vi "S4GUI.vi"() -> ()   [LabVIEW 2018] (continued)
  T9 = cluster{"Trigger Mode Status":string, "String output":string, "Instrument Status":cluster{"WPROT pos":dbl, "WPSEL pos":dbl, "GMIR pos":dbl, "GFOC pos":dbl, "CALW pos":dbl, "ASEL pos":dbl, "connection":bool, "mode":bool, "String Status":string}, "Sync Box State":i32, "Trigger General Status":string, "Instrument States":cluster{"WPSEL State":i32, "WPROT State":i32, "CALW State":i32, "ASEL State":i32, "GMIR State":i32, "GFOC State":i32}, "Instrument Pos Names":cluster{"WPROT posname":string, "WPSEL posname":string, "CALW posname":string, "ASEL posname":string}, "ChannelA_Status":cluster{"Current exp":dbl, "Frames done":u32, "LastFileImage":string, "CamStatus":string, "Run state":u32, "connection":bool, "Cooler ON/OFF":i16, "Currently temperature":i16, "Temperature Status":string, "target  temp":i16, "conf runing":bool}, "WPROT seq":u16, "ChannelB_Status":cluster{"Current exp":dbl, "Frames done":u32, "LastFileImage":string, "CamStatus":string, "Run state":u32, "connection":bool, "Cooler ON/OFF":i16, "Currently temperature":i16, "Temperature Status":string, "target  temp":i16, "conf runing":bool}, "ChannelC_Status":cluster{"Current exp":dbl, "Frames done":u32, "LastFileImage":string, "CamStatus":string, "Run state":u32, "connection":bool, "Cooler ON/OFF":i16, "Currently temperature":i16, "Temperature Status":string, "target  temp":i16, "conf runing":bool}, "ChannelD_Status":cluster{"Current exp":dbl, "Frames done":u32, "LastFileImage":string, "CamStatus":string, "Run state":u32, "connection":bool, "Cooler ON/OFF":i16, "Currently temperature":i16, "Temperature Status":string, "target  temp":i16, "conf runing":bool}, "ChannelA_CCD":cluster{"ACQUISITION_MODE":u8, "TRIGGER_MODE":u8, "READ_MODE":u8, "PREAMP":u8, "READOUT_RATE":u8, "VERTICAL_SHIFT_SPEED":u8, "EM_MODE":u8, "EM_GAIN":u16, "SHUTTER_MODE":u8, "SHUTTER_TTL":u8, "SHUTTER_OPENNING_TIME":u16, "SHUTTER_CLOSING_TIME":u16, "VBIN":u16, "HBIN":u16, "INITIAL_LINE":u16, "INITIAL_COLUMN":u16, "FINAL_LINE":u16, "FINAL_COLUMN":u16, "FRAME_TRANSFER":bool, "VERTICAL_CLOCK_VOLTAGE":u8, "AD_CHANNEL":u32}, "ChannelB_CCD ":cluster{"ACQUISITION_MODE":u8, "TRIGGER_MODE":u8, "READ_MODE":u8, "PREAMP":u8, "READOUT_RATE":u8, "VERTICAL_SHIFT_SPEED":u8, "EM_MODE":u8, "EM_GAIN":u16, "SHUTTER_MODE":u8, "SHUTTER_TTL":u8, "SHUTTER_OPENNING_TIME":u16, "SHUTTER_CLOSING_TIME":u16, "VBIN":u16, "HBIN":u16, "INITIAL_LINE":u16, "INITIAL_COLUMN":u16, "FINAL_LINE":u16, "FINAL_COLUMN":u16, "FRAME_TRANSFER":bool, "VERTICAL_CLOCK_VOLTAGE":u8, "AD_CHANNEL":u32}, "ChannelC_CCD":cluster{"ACQUISITION_MODE":u8, "TRIGGER_MODE":u8, "READ_MODE":u8, "PREAMP":u8, "READOUT_RATE":u8, "VERTICAL_SHIFT_SPEED":u8, "EM_MODE":u8, "EM_GAIN":u16, "SHUTTER_MODE":u8, "SHUTTER_TTL":u8, "SHUTTER_OPENNING_TIME":u16, "SHUTTER_CLOSING_TIME":u16, "VBIN":u16, "HBIN":u16, "INITIAL_LINE":u16, "INITIAL_COLUMN":u16, "FINAL_LINE":u16, "FINAL_COLUMN":u16, "FRAME_TRANSFER":bool, "VERTICAL_CLOCK_VOLTAGE":u8, "AD_CHANNEL":u32}, "ChannelD_CCD":cluster{"ACQUISITION_MODE":u8, "TRIGGER_MODE":u8, "READ_MODE":u8, "PREAMP":u8, "READOUT_RATE":u8, "VERTICAL_SHIFT_SPEED":u8, "EM_MODE":u8, "EM_GAIN":u16, "SHUTTER_MODE":u8, "SHUTTER_TTL":u8, "SHUTTER_OPENNING_TIME":u16, "SHUTTER_CLOSING_TIME":u16, "VBIN":u16, "HBIN":u16, "INITIAL_LINE":u16, "INITIAL_COLUMN":u16, "FINAL_LINE":u16, "FINAL_COLUMN":u16, "FRAME_TRANSFER":bool, "VERTICAL_CLOCK_VOLTAGE":u8, "AD_CHANNEL":u32}, "CHA_Checked Params":cluster{"ACQUISITION_MODE":bool, "TRIGGER_MODE":bool, "READ_MODE":bool, "PREAMP":bool, "READOUT_RATE":bool, "VERTICAL_SHIFT_SPEED":bool, "EM_MODE":bool, "EM_GAIN":bool, "SHUTTER_MODE":bool, "SHUTTER_TTL":bool, "SHUTTER_OPENING_TIME":bool, "SHUTTER_CLOSING_TIME":bool, "VBIN":bool, "HBIN":bool, "INITIAL_LINE":bool, "INITIAL_COLUMN":bool, "FINAL_LINE":bool, "FINAL_COLUMN":bool, "FRAME_TRANSFER":bool, "VERTICAL_CLOCK_VOLTAGE":bool, "AD_CHANNEL":bool}, "CHB_Checked Params":cluster{"ACQUISITION_MODE":bool, "TRIGGER_MODE":bool, "READ_MODE":bool, "PREAMP":bool, "READOUT_RATE":bool, "VERTICAL_SHIFT_SPEED":bool, "EM_MODE":bool, "EM_GAIN":bool, "SHUTTER_MODE":bool, "SHUTTER_TTL":bool, "SHUTTER_OPENING_TIME":bool, "SHUTTER_CLOSING_TIME":bool, "VBIN":bool, "HBIN":bool, "INITIAL_LINE":bool, "INITIAL_COLUMN":bool, "FINAL_LINE":bool, "FINAL_COLUMN":bool, "FRAME_TRANSFER":bool, "VERTICAL_CLOCK_VOLTAGE":bool, "AD_CHANNEL":bool}, "CHC_Checked Params":cluster{"ACQUISITION_MODE":bool, "TRIGGER_MODE":bool, "READ_MODE":bool, "PREAMP":bool, "READOUT_RATE":bool, "VERTICAL_SHIFT_SPEED":bool, "EM_MODE":bool, "EM_GAIN":bool, "SHUTTER_MODE":bool, "SHUTTER_TTL":bool, "SHUTTER_OPENING_TIME":bool, "SHUTTER_CLOSING_TIME":bool, "VBIN":bool, "HBIN":bool, "INITIAL_LINE":bool, "INITIAL_COLUMN":bool, "FINAL_LINE":bool, "FINAL_COLUMN":bool, "FRAME_TRANSFER":bool, "VERTICAL_CLOCK_VOLTAGE":bool, "AD_CHANNEL":bool}, "CHD_Checked Params":cluster{"ACQUISITION_MODE":bool, "TRIGGER_MODE":bool, "READ_MODE":bool, "PREAMP":bool, "READOUT_RATE":bool, "VERTICAL_SHIFT_SPEED":bool, "EM_MODE":bool, "EM_GAIN":bool, "SHUTTER_MODE":bool, "SHUTTER_TTL":bool, "SHUTTER_OPENING_TIME":bool, "SHUTTER_CLOSING_TIME":bool, "VBIN":bool, "HBIN":bool, "INITIAL_LINE":bool, "INITIAL_COLUMN":bool, "FINAL_LINE":bool, "FINAL_COLUMN":bool, "FRAME_TRANSFER":bool, "VERTICAL_CLOCK_VOLTAGE":bool, "AD_CHANNEL":bool}, "Trigger_connection":bool, "TCSPD_connection":bool, "TCS extended":string}
  T10 = cluster{"Cluster Mode Sync":cluster{"#Index Cycles":enum8{"Enabled", "Disabled", "Disabled and Grayed Out"}, "#Cycles":enum8{"Enabled", "Disabled", "Disabled and Grayed Out"}, "SSM":enum8{"Enabled", "Disabled", "Disabled and Grayed Out"}, "Set SM":enum8{"Enabled", "Disabled", "Disabled and Grayed Out"}, "Star SM":enum8{"Enabled", "Disabled", "Disabled and Grayed Out"}, "Pause SM":enum8{"Enabled", "Disabled", "Disabled and Grayed Out"}, "Stop SM":enum8{"Enabled", "Disabled", "Disabled and Grayed Out"}, "Abort SM":enum8{"Enabled", "Disabled", "Disabled and Grayed Out"}, "Start SM Text":string}, "Cluster Polarimetry":cluster{"Lambda Selector":enum8{"Enabled", "Disabled", "Disabled and Grayed Out"}, "Calibrator Selector":enum8{"Enabled", "Disabled", "Disabled and Grayed Out"}, "Set Waveplate":enum8{"Enabled", "Disabled", "Disabled and Grayed Out"}, "Select Positions":enum8{"Enabled", "Disabled", "Disabled and Grayed Out"}, "P0":enum8{"Enabled", "Disabled", "Disabled and Grayed Out"}, "P1":enum8{"Enabled", "Disabled", "Disabled and Grayed Out"}, "P2":enum8{"Enabled", "Disabled", "Disabled and Grayed Out"}, "P3":enum8{"Enabled", "Disabled", "Disabled and Grayed Out"}, "P4":enum8{"Enabled", "Disabled", "Disabled and Grayed Out"}, "P5":enum8{"Enabled", "Disabled", "Disabled and Grayed Out"}, "P6":enum8{"Enabled", "Disabled", "Disabled and Grayed Out"}, "P7":enum8{"Enabled", "Disabled", "Disabled and Grayed Out"}, "P8":enum8{"Enabled", "Disabled", "Disabled and Grayed Out"}, "P9":enum8{"Enabled", "Disabled", "Disabled and Grayed Out"}, "P10":enum8{"Enabled", "Disabled", "Disabled and Grayed Out"}, "P11":enum8{"Enabled", "Disabled", "Disabled and Grayed Out"}, "P12":enum8{"Enabled", "Disabled", "Disabled and Grayed Out"}, "P13":enum8{"Enabled", "Disabled", "Disabled and Grayed Out"}, "P14":enum8{"Enabled", "Disabled", "Disabled and Grayed Out"}, "P15":enum8{"Enabled", "Disabled", "Disabled and Grayed Out"}}, "Cluster Mode CH1":cluster{"#cycles ch1":enum8{"Enabled", "Disabled", "Disabled and Grayed Out"}, "Start ch1":enum8{"Enabled", "Disabled", "Disabled and Grayed Out"}, "Pause ch1":enum8{"Enabled", "Disabled", "Disabled and Grayed Out"}, "Stop ch1":enum8{"Enabled", "Disabled", "Disabled and Grayed Out"}, "Abort ch1":enum8{"Enabled", "Disabled", "Disabled and Grayed Out"}, "Exptime ch1":enum8{"Enabled", "Disabled", "Disabled and Grayed Out"}, "Exp ch1":enum8{"Enabled", "Disabled", "Disabled and Grayed Out"}, "Start ch1 Text":string, "Set Cooler":enum8{"Enabled", "Disabled", "Disabled and Grayed Out"}, "Set Temp":enum8{"Enabled", "Disabled", "Disabled and Grayed Out"}}, "Cluster Mode CH2":cluster{"#cycles ch2":enum8{"Enabled", "Disabled", "Disabled and Grayed Out"}, "Start ch2":enum8{"Enabled", "Disabled", "Disabled and Grayed Out"}, "Pause ch2":enum8{"Enabled", "Disabled", "Disabled and Grayed Out"}, "Stop ch2":enum8{"Enabled", "Disabled", "Disabled and Grayed Out"}, "Abort ch2":enum8{"Enabled", "Disabled", "Disabled and Grayed Out"}, "Exptime ch2":enum8{"Enabled", "Disabled", "Disabled and Grayed Out"}, "Exp ch2":enum8{"Enabled", "Disabled", "Disabled and Grayed Out"}, "Start ch2 Text":string, "Set Cooler":enum8{"Enabled", "Disabled", "Disabled and Grayed Out"}, "Set Temp":enum8{"Enabled", "Disabled", "Disabled and Grayed Out"}}, "Cluster Mode CH3":cluster{"#cycles ch3":enum8{"Enabled", "Disabled", "Disabled and Grayed Out"}, "Start ch3":enum8{"Enabled", "Disabled", "Disabled and Grayed Out"}, "Pause ch3":enum8{"Enabled", "Disabled", "Disabled and Grayed Out"}, "Stop ch3":enum8{"Enabled", "Disabled", "Disabled and Grayed Out"}, "Abort ch3":enum8{"Enabled", "Disabled", "Disabled and Grayed Out"}, "Exptime ch3":enum8{"Enabled", "Disabled", "Disabled and Grayed Out"}, "Exp ch3":enum8{"Enabled", "Disabled", "Disabled and Grayed Out"}, "Start ch3 Text":string, "Set Cooler":enum8{"Enabled", "Disabled", "Disabled and Grayed Out"}, "Set Temp":enum8{"Enabled", "Disabled", "Disabled and Grayed Out"}}, "Cluster Mode CH4":cluster{"#cycles ch4":enum8{"Enabled", "Disabled", "Disabled and Grayed Out"}, "Start ch4":enum8{"Enabled", "Disabled", "Disabled and Grayed Out"}, "Pause ch4":enum8{"Enabled", "Disabled", "Disabled and Grayed Out"}, "Stop ch4":enum8{"Enabled", "Disabled", "Disabled and Grayed Out"}, "Abort ch4":enum8{"Enabled", "Disabled", "Disabled and Grayed Out"}, "Exptime ch4":enum8{"Enabled", "Disabled", "Disabled and Grayed Out"}, "Exp ch4":enum8{"Enabled", "Disabled", "Disabled and Grayed Out"}, "Start ch4 Text":string, "Set Cooler":enum8{"Enabled", "Disabled", "Disabled and Grayed Out"}, "Set Temp":enum8{"Enabled", "Disabled", "Disabled and Grayed Out"}}, "Cluster ExpMode":cluster{"tab4":enum8{"Enabled", "Disabled", "Disabled and Grayed Out"}}}
  T11 = cluster{"WPROT pos":dbl, "WPSEL pos":dbl, "GMIR pos":dbl, "GFOC pos":dbl, "CALW pos":dbl, "ASEL pos":dbl, "connection":bool, "mode":bool, "String Status":string}
  T12 = cluster{"WPSEL State":i32, "WPROT State":i32, "CALW State":i32, "ASEL State":i32, "GMIR State":i32, "GFOC State":i32}
  T13 = cluster{"WPROT posname":string, "WPSEL posname":string, "CALW posname":string, "ASEL posname":string}
  T14 = cluster{"Current exp":dbl, "Frames done":u32, "LastFileImage":string, "CamStatus":string, "Run state":u32, "connection":bool, "Cooler ON/OFF":i16, "Currently temperature":i16, "Temperature Status":string, "target  temp":i16, "conf runing":bool}
  T15 = cluster{"Lambda Selector":enum8{"Enabled", "Disabled", "Disabled and Grayed Out"}, "Calibrator Selector":enum8{"Enabled", "Disabled", "Disabled and Grayed Out"}, "Set Waveplate":enum8{"Enabled", "Disabled", "Disabled and Grayed Out"}, "Select Positions":enum8{"Enabled", "Disabled", "Disabled and Grayed Out"}, "P0":enum8{"Enabled", "Disabled", "Disabled and Grayed Out"}, "P1":enum8{"Enabled", "Disabled", "Disabled and Grayed Out"}, "P2":enum8{"Enabled", "Disabled", "Disabled and Grayed Out"}, "P3":enum8{"Enabled", "Disabled", "Disabled and Grayed Out"}, "P4":enum8{"Enabled", "Disabled", "Disabled and Grayed Out"}, "P5":enum8{"Enabled", "Disabled", "Disabled and Grayed Out"}, "P6":enum8{"Enabled", "Disabled", "Disabled and Grayed Out"}, "P7":enum8{"Enabled", "Disabled", "Disabled and Grayed Out"}, "P8":enum8{"Enabled", "Disabled", "Disabled and Grayed Out"}, "P9":enum8{"Enabled", "Disabled", "Disabled and Grayed Out"}, "P10":enum8{"Enabled", "Disabled", "Disabled and Grayed Out"}, "P11":enum8{"Enabled", "Disabled", "Disabled and Grayed Out"}, "P12":enum8{"Enabled", "Disabled", "Disabled and Grayed Out"}, "P13":enum8{"Enabled", "Disabled", "Disabled and Grayed Out"}, "P14":enum8{"Enabled", "Disabled", "Disabled and Grayed Out"}, "P15":enum8{"Enabled", "Disabled", "Disabled and Grayed Out"}}
  T16 = cluster{"#Index Cycles":enum8{"Enabled", "Disabled", "Disabled and Grayed Out"}, "#Cycles":enum8{"Enabled", "Disabled", "Disabled and Grayed Out"}, "SSM":enum8{"Enabled", "Disabled", "Disabled and Grayed Out"}, "Set SM":enum8{"Enabled", "Disabled", "Disabled and Grayed Out"}, "Star SM":enum8{"Enabled", "Disabled", "Disabled and Grayed Out"}, "Pause SM":enum8{"Enabled", "Disabled", "Disabled and Grayed Out"}, "Stop SM":enum8{"Enabled", "Disabled", "Disabled and Grayed Out"}, "Abort SM":enum8{"Enabled", "Disabled", "Disabled and Grayed Out"}, "Start SM Text":string}
  T17 = cluster{"#cycles ch1":enum8{"Enabled", "Disabled", "Disabled and Grayed Out"}, "Start ch1":enum8{"Enabled", "Disabled", "Disabled and Grayed Out"}, "Pause ch1":enum8{"Enabled", "Disabled", "Disabled and Grayed Out"}, "Stop ch1":enum8{"Enabled", "Disabled", "Disabled and Grayed Out"}, "Abort ch1":enum8{"Enabled", "Disabled", "Disabled and Grayed Out"}, "Exptime ch1":enum8{"Enabled", "Disabled", "Disabled and Grayed Out"}, "Exp ch1":enum8{"Enabled", "Disabled", "Disabled and Grayed Out"}, "Start ch1 Text":string, "Set Cooler":enum8{"Enabled", "Disabled", "Disabled and Grayed Out"}, "Set Temp":enum8{"Enabled", "Disabled", "Disabled and Grayed Out"}}
  T18 = cluster{"#cycles ch2":enum8{"Enabled", "Disabled", "Disabled and Grayed Out"}, "Start ch2":enum8{"Enabled", "Disabled", "Disabled and Grayed Out"}, "Pause ch2":enum8{"Enabled", "Disabled", "Disabled and Grayed Out"}, "Stop ch2":enum8{"Enabled", "Disabled", "Disabled and Grayed Out"}, "Abort ch2":enum8{"Enabled", "Disabled", "Disabled and Grayed Out"}, "Exptime ch2":enum8{"Enabled", "Disabled", "Disabled and Grayed Out"}, "Exp ch2":enum8{"Enabled", "Disabled", "Disabled and Grayed Out"}, "Start ch2 Text":string, "Set Cooler":enum8{"Enabled", "Disabled", "Disabled and Grayed Out"}, "Set Temp":enum8{"Enabled", "Disabled", "Disabled and Grayed Out"}}
  T19 = cluster{"#cycles ch3":enum8{"Enabled", "Disabled", "Disabled and Grayed Out"}, "Start ch3":enum8{"Enabled", "Disabled", "Disabled and Grayed Out"}, "Pause ch3":enum8{"Enabled", "Disabled", "Disabled and Grayed Out"}, "Stop ch3":enum8{"Enabled", "Disabled", "Disabled and Grayed Out"}, "Abort ch3":enum8{"Enabled", "Disabled", "Disabled and Grayed Out"}, "Exptime ch3":enum8{"Enabled", "Disabled", "Disabled and Grayed Out"}, "Exp ch3":enum8{"Enabled", "Disabled", "Disabled and Grayed Out"}, "Start ch3 Text":string, "Set Cooler":enum8{"Enabled", "Disabled", "Disabled and Grayed Out"}, "Set Temp":enum8{"Enabled", "Disabled", "Disabled and Grayed Out"}}
  T20 = cluster{"#cycles ch4":enum8{"Enabled", "Disabled", "Disabled and Grayed Out"}, "Start ch4":enum8{"Enabled", "Disabled", "Disabled and Grayed Out"}, "Pause ch4":enum8{"Enabled", "Disabled", "Disabled and Grayed Out"}, "Stop ch4":enum8{"Enabled", "Disabled", "Disabled and Grayed Out"}, "Abort ch4":enum8{"Enabled", "Disabled", "Disabled and Grayed Out"}, "Exptime ch4":enum8{"Enabled", "Disabled", "Disabled and Grayed Out"}, "Exp ch4":enum8{"Enabled", "Disabled", "Disabled and Grayed Out"}, "Start ch4 Text":string, "Set Cooler":enum8{"Enabled", "Disabled", "Disabled and Grayed Out"}, "Set Temp":enum8{"Enabled", "Disabled", "Disabled and Grayed Out"}}
  T21 = cluster{"ACQUISITION_MODE":u8, "TRIGGER_MODE":u8, "READ_MODE":u8, "PREAMP":u8, "READOUT_RATE":u8, "VERTICAL_SHIFT_SPEED":u8, "EM_MODE":u8, "EM_GAIN":u16, "SHUTTER_MODE":u8, "SHUTTER_TTL":u8, "SHUTTER_OPENNING_TIME":u16, "SHUTTER_CLOSING_TIME":u16, "VBIN":u16, "HBIN":u16, "INITIAL_LINE":u16, "INITIAL_COLUMN":u16, "FINAL_LINE":u16, "FINAL_COLUMN":u16, "FRAME_TRANSFER":bool, "VERTICAL_CLOCK_VOLTAGE":u8, "AD_CHANNEL":u32}
  T22 = cluster{"ACQUISITION_MODE":bool, "TRIGGER_MODE":bool, "READ_MODE":bool, "PREAMP":bool, "READOUT_RATE":bool, "VERTICAL_SHIFT_SPEED":bool, "EM_MODE":bool, "EM_GAIN":bool, "SHUTTER_MODE":bool, "SHUTTER_TTL":bool, "SHUTTER_OPENING_TIME":bool, "SHUTTER_CLOSING_TIME":bool, "VBIN":bool, "HBIN":bool, "INITIAL_LINE":bool, "INITIAL_COLUMN":bool, "FINAL_LINE":bool, "FINAL_COLUMN":bool, "FRAME_TRANSFER":bool, "VERTICAL_CLOCK_VOLTAGE":bool, "AD_CHANNEL":bool}
  T23 = cluster{"Image \nInitial Line":u16, "Image\nInitial Column":u16, "Image\nFinal Line":u16, "Image\nFInal Column":u16, "Vertical\nBinning":u16, "Horizontal\nBinning":u16, "Pre-amplification\nGain":u8, "CCD\nEM Gain":u16, "Readout\nRate":u8, "Shutter\nOpenning Time":i32, "Shutter\nClosing Time":i32, "Vertical\nShift Speed":u8, "Read\nMode":u8, "Vertical\nClock Voltage":u8, "A/D \nChannel":u32, "Shutter\nMode":u16, "Shutter\nTTL":u16, "Trigger\nMode":u16, "Frame\nTransfer":bool, "Acquisition\nMode":u8, "CCD \nEM Mode":u8}
  T24 = cluster{"ACQUISITION_MODE":u8, "TRIGGER_MODE":u8, "READ_MODE":u8, "PREAMP":u8, "READOUT_RATE":u8, "VERTICAL_SHIFT_SPEED":u8, "EM_MODE":u8, "EM_GAIN":u16, "SHUTTER_MODE":u8, "SHUTTER_TTL":u8, "SHUTTER_OPENING_TIME":u16, "SHUTTER_CLOSING_TIME":u16, "VBIN":u16, "HBIN":u16, "INITIAL_LINE":u16, "INITIAL_COLUMN":u16, "FINAL_LINE":u16, "FINAL_COLUMN":u16, "FRAME_TRANSFER":bool, "VERTICAL_CLOCK_VOLTAGE":u8, "AD_CHANNEL":u32}
  T25 = cluster{"Image Initial Line":dbl, "Image Initial Column":dbl, "Image Final Line":dbl, "Image FInal Column":dbl, "Vertical Binning":dbl, "Horizontal Binning":dbl, "Pre-amplification Gain":u8, "CCD EM Gain":u8, "Readout Rate":u8, "Shutter Openning Time":i32, "Shutter Closing Time":i32, "Vertical Shift Speed":u8, "Read Mode":u8, "Vertical Clock Voltage":u8, "A/D  Channel":u32, "Image Initial Line 2":dbl, "Image Initial Column 2":dbl, "Image Final Line 2":dbl, "Image FInal Column 2":dbl, "Vertical Binning 2":dbl, "Horizontal Binning 2":dbl, "Pre-amplification Gain 2":u8, "CCD EM Gain 2":u16, "Readout Rate 2":u8, "Shutter Openning Time 2":i32, "Shutter Closing Time 2":i32, "Vertical Shift Speed 2":u8, "Read Mode 2":u8, "Vertical Clock Voltage 2":u8, "A/D Channel 2":u32, "Image Initial Line 3":dbl, "Image Initial Column 3":dbl, "Image Final Line 3":dbl, "Image FInal Column 3":dbl, "Vertical Binning 3":dbl, "Horizontal Binning 3":dbl, "Pre-amplification Gain 3":u8, "CCD EM Gain 3":u16, "Readout Rate 3":u8, "Shutter Openning Time 3":i32, "Shutter Closing Time 3":i32, "Vertical Shift Speed 3":u8, "Read Mode 3":u8, "Vertical Clock Voltage 3":u8, "A/D Channel 3":u32, "Image Initial Line 4":dbl, "Image Initial Column 4":dbl, "Image Final Line 4":dbl, "Image FInal Column 4":dbl, "Vertical Binning 4":dbl, "Horizontal Binning 4":dbl, "Pre-amplification Gain 4":u8, "CCD EM Gain 4":u16, "Readout Rate 4":u8, "Shutter Openning Time 4":i32, "Shutter Closing Time 4":i32, "Vertical Shift Speed 4":u8, "Read Mode 4":u8, "Vertical Clock Voltage 4":u8, "A/D Channel 4":u32, "CCD EM Mode 2":u8, "CCD EM Mode 3":u8, "CCD EM Mode 4":u8, "CCD EM Mode":u16, "Shutter Mode":u16, "Shutter Mode 2":u16, "Shutter Mode 4":u16, "Shutter Mode 3":u16, "Shutter TTL":u16, "Shutter TTL 2":u16, "Shutter TTL 3":u16, "Shutter TTL 4":u16, "Frame Transfer":bool, "Frame Transfer 2":bool, "Frame Transfer 3":bool, "Frame Transfer 4":bool, "Trigger Mode":u16, "Trigger Mode 2":u16, "Trigger Mode 3":u16, "Trigger Mode 4":u16, "Acquisition Mode":u8, "Acquisition Mode 2":u8, "Acquisition Mode 3":u8, "Acquisition Mode 4":u8}
diagram:
  w5 = T7."Disabled" ("Disabled")
  (unwired) -400 ("Position:Top")
  w10 = "" ("Temp Status 1")
  w11 = i16 0 ("Curr Temp 1")
  w12 = FALSE ("Cooler status 1")
  w13 = u16 1 items=["Asynchronous", "Synchronous by Cycle"] ("SSM")
  (unwired) -400 ("Position:Top")
  w25 = u16 4 items=["All 16 positions", "First 8 positions", "First 4 positions", "1-4 & 9-12", "Clear", "Customized"] ("Select Positions")
  w4 = FALSE
  n1 = local write "Select Positions"(w25) -> ()
  n2 = property on="Tab Acq Type" class="TabCtl (strict)"("DisabledEnum"=T7."Disabled and Grayed Out" ("Disabled")) -> ()  [unwired: 2 in, 2 out]
  n3 = property on="Tab ObsEng" class="TabCtl (strict)"("Visible"=TRUE) -> ()  [unwired: 2 in, 2 out]
  n4 = flat-sequence {
    tunnel: errorcluster {"status"=FALSE, "code"=0, "source"=""} ("error in (no error)") -> [w30]
    tunnel: [w30] -> w7
    frame #0 {
      w31 = u32 240 ("Tab Control Pane Dimension:Width")
      w32 = u32 300 ("Tab Control Pane Dimension:Height")
      n5 = property on="Tab CH2" class="TabCtl (strict)"("PaneHeight"=w32, "PaneWidth"=w31) -> ()  [unwired: 2 in, 2 out]
      n6 = property on="Tab CH1" class="TabCtl (strict)"("PaneHeight"=w32, "PaneWidth"=w31) -> ()  [unwired: 2 in, 2 out]
      n7 = property on="Tab CH3" class="TabCtl (strict)"("PaneHeight"=w32, "PaneWidth"=w31) -> ()  [unwired: 2 in, 2 out]
      n8 = property on="Tab CH4" class="TabCtl (strict)"("PaneHeight"=w32, "PaneWidth"=w31) -> ()  [unwired: 2 in, 2 out]
      n9 = local write "loop max(ms)"(u32 0 ("loop max(ms)")) -> ()
    }
  }
  n10 = property on="SSM" class="Ring (strict)"("Value"=w13) -> ()  [unwired: 2 in, 2 out]
  n11 = disable-structure shown="Enabled" {
    disable-tunnel: "S4ACS_GUI.lvclass" -> [w41 w42]
    disable-tunnel: [w38 w42] -> w16
    disable-tunnel: w7 -> [w40 w43]
    disable-tunnel: [w39 w43] -> w15
    frame Enabled {
      # "Carrega o ultimo filtro escolhido para os 4 canais."
      n12 = local read "Filter1"() -> (w37:u8)
      n13 = local read "Filter2"() -> (w36:u8)
      n14 = local read "Filter3"() -> (w35:u8)
      n15 = local read "Filter4"() -> (w34:u8)
      n16 = call-dynamic "LoadFilters.vi"("Filter 4"=w34, "Filter 3"=w35, "error in (no error)"=w40, "Filter 2"=w36, "Filter 1"=w37, "S4GUI in"=w41) -> ("error out"=w39:errorcluster, "S4GUI out"=w38:refnum<class "S4GUI.lvclass">)  [unwired: 4 in]
    }
    frame Disabled {
    }
  }
  n17 = flat-sequence "Indicadores dos canais da parte inferior da tela principal" {
    frame #0 {
      w44 = ""
      "B1" <- w44
      "PA1" <- w44
      "RO1" <- w44
      "G1" <- w44
      "SI2" <- w44
      "PA2" <- w44
      "G2" <- w44
      "B2" <- w44
      "RO2" <- w44
      "EA2" <- w44
      "SI3" <- w44
      "EA3" <- w44
      "PA3" <- w44
      "B3" <- w44
      "G3" <- w44
      "RO3" <- w44
      "SI4" <- w44
      "EA4" <- w44
      "PA4" <- w44
      "B4" <- w44
      "G4" <- w44
      "RO4" <- w44
      "SI1" <- w44
      "EA1" <- w44
    }
  }
  n18 = local write "Cooler status 4"(w12) -> ()
  n19 = local write "Curr Temp 4"(w11) -> ()
  n20 = local write "Panel Temp 4"(w11) -> ()
  n21 = local write "Temp Status 4"(w10) -> ()
  n22 = local write "Panel cooler 4"(w12) -> ()
  n23 = local write "Cooler status 1"(w12) -> ()
  n24 = local write "Curr Temp 1"(w11) -> ()
  n25 = local write "Panel Temp"(w11) -> ()
  n26 = local write "Temp Status 1"(w10) -> ()
  n27 = local write "Panel cooler 2"(w12) -> ()
  n28 = local write "Curr Temp 2"(w11) -> ()
  n29 = local write "Panel Temp 2"(w11) -> ()
  n30 = local write "Temp Status 2"(w10) -> ()
  n31 = local write "Panel cooler 3"(w12) -> ()
  n32 = local write "Cooler status 3"(w12) -> ()
  n33 = local write "Curr Temp 3"(w11) -> ()
  n34 = local write "Panel Temp 3"(w11) -> ()
  n35 = local write "Temp Status 3"(w10) -> ()
  n36 = control-ref of="Current Configuration"() -> (w23:refnum<vi>)
  n37 = local write "Cooler status 2"(w12) -> ()
  n38 = control-ref of="Parameters"() -> (w19:refnum<vi>)
  n39 = local write "Cooler"(w12) -> ()
  n40 = property on="Property Node" class="Clust (strict)"(reference=w19, "Top"=-580 ("Position:Top")) -> (reference out=w24:refnum<vi>)  [unwired: 1 in, 1 out]
  n41 = property on="Property Node" class="Clust (strict)"(reference=w23, "Top"=-580 ("Position:Top")) -> (reference out=w22:refnum<vi>)  [unwired: 1 in, 1 out]
  n42 = disable-structure shown="Enabled" {
    frame Enabled {
      n43 = property on="Observer" class="Str"("Value"="" ("Observer"), "Text.BGColor"=u32 16448250) -> ()  [unwired: 2 in, 2 out]
    }
    frame Disabled {
    }
  }
  n44 = property on="ExtSync" class="Bool (strict)"("Value"=TRUE ("ExtSync")) -> ()  [unwired: 2 in, 2 out]
  n45 = local write "GUIDER"(FALSE ("GUIDER")) -> ()
  n46 = local write "rotator"(0.0 ("rotator")) -> ()
  n47 = property on="Object_dflat" class="Str"("DisabledEnum"=w5) -> ()  [unwired: 2 in, 2 out]
  n48 = property on="Object_zero" class="Str"("DisabledEnum"=w5) -> ()  [unwired: 2 in, 2 out]
  n49 = property on="Object_sflat" class="Str"("DisabledEnum"=w5) -> ()  [unwired: 2 in, 2 out]
  n50 = Bundle("Parameters"=w24, "Current Configuration"=w22) -> (w20:T8)  [unwired: 1 in]
  n51 = call-dynamic "Initialize.vi"("error in (no error)"=w15, "S4ACS_GUI in"=w16) -> ("error out"=w28:errorcluster, "S4ACS_GUI out"=w29:refnum<class "S4GUI.lvclass">)  [unwired: 8 in]
  n52 = local write "P8"(w4) -> ()
  n53 = local write "P9"(w4) -> ()
  n54 = local write "P10"(w4) -> ()
  n55 = local write "P11"(w4) -> ()
  n56 = local write "P12"(w4) -> ()
  n57 = local write "P13"(w4) -> ()
  n58 = local write "P14"(w4) -> ()
  n59 = local write "P15"(w4) -> ()
  n60 = local write "P1"(w4) -> ()
  n61 = local write "P2"(w4) -> ()
  n62 = local write "P3"(w4) -> ()
  n63 = local write "P4"(w4) -> ()
  n64 = local write "P5"(w4) -> ()
  n65 = local write "P6"(w4) -> ()
  n66 = local write "P7"(w4) -> ()
  n67 = local write "P0"(TRUE ("P0")) -> ()
  n68 = while {
    shift-right: [w54] -> w27
    shift-left: w29 -> [w57]
    shift-right: [w67] -> _
    shift-left: w28 -> [w68]
    tunnel: w20 -> [w62]
    stop <- w66 stop-if-true
    # "Sufixo do arquivo SEMPRE\nem minúsculas."
    n69 = case shown="\"OBJECT\", Default" "Tab Acq Type" {
      tunnel: ["object suffix" "dflat suffix" "sflat suffix" "dark suffix" "zero suffix" "focus suffix"] -> w49
      tunnel: ["OBJECT Comments" "DFLAT Comments" "SFLAT Comments" "DARK Comments" "ZERO Comments" "FOCUS Comments"] -> w63
      tunnel: ["OBJECT" "FLAT" "FLAT" "DARK" "ZERO" "FOCUS"] -> w60
      tunnel: ["Object_obj" "DOMEFLAT" "SKYFLAT" "Object_dark" "ZERO" "Object_focus"] -> w59
      frame "OBJECT", Default {
      }
      frame "DFLAT" {
      }
      frame "SFLAT" {
      }
      frame "DARK" {
      }
      frame "ZERO" {
      }
      frame "FOCUS" {
      }
    }
    n70 = flat-sequence {
      tunnel: w57 -> [w81]
      tunnel: [w81] -> w56
      tunnel: [w80] -> w53
      frame #0 {
        n71 = case shown="True" "reset max" {
          frame False {
          }
          frame True {
            n72 = local write "loop max(ms)"(u32 0 ("loop max(ms)")) -> ()
          }
        }
        n73 = Tick Count (ms)() -> (millisecond timer value=w80:u32)
      }
    }
    n74 = To Lower Case(string=w49) -> (all lower case string=w48:string)
    n75 = event shown="[23] \"# Cycles\": Value Change" {
      selector: _ -> [_ _ _ _ _ _ _ _ _ _ _ _ _ _ _ _ _ _ _ _ _ _ _ _ _ _ _ _ _ _ _ _ _ _ _ _ _ _ _ _ _ _ _ _ _ _ _ _ _ _ _ _ _ _ _ _ _ _ _ _ _ _ _ _ _ _ _ _ _ _ _ _ _ _ _ _ _ _ _ _ _ _ _ _ _ _ _ _ _ _ _ _ _ _ _ _ _ _ _ _ _ _ _ _ _ _ _ _ _]
      dyn-events: _ -> [_ _ _ _ _ _ _ _ _ _ _ _ _ _ _ _ _ _ _ _ _ _ _ _ _ _ _ _ _ _ _ _ _ _ _ _ _ _ _ _ _ _ _ _ _ _ _ _ _ _ _ _ _ _ _ _ _ _ _ _ _ _ _ _ _ _ _ _ _ _ _ _ _ _ _ _ _ _ _ _ _ _ _ _ _ _ _ _ _ _ _ _ _ _ _ _ _ _ _ _ _ _ _ _ _ _ _ _ _]
      timeout: 20 -> [_ _ _ _ _ _ _ _ _ _ _ _ _ _ _ _ _ _ _ _ _ _ _ _ _ _ _ _ _ _ _ _ _ _ _ _ _ _ _ _ _ _ _ _ _ _ _ _ _ _ _ _ _ _ _ _ _ _ _ _ _ _ _ _ _ _ _ _ _ _ _ _ _ _ _ _ _ _ _ _ _ _ _ _ _ _ _ _ _ _ _ _ _ _ _ _ _ _ _ _ _ _ _ _ _ _ _ _ _]
      tunnel: w56 -> [w137 w1481 w1557 w1641 w1708 w1775 w1807 w1822 w1948 w2127 w2159 w2191 w2223 w2257 w2291 w2325 w2362 w2365 w2399 w2541 w2594 w3155 w3213 w3574 w3581 w3671 w4398 w4579 w4768 w4951 w5146 w5154 w5163 w5343 w5465 w5589 w5714 w5834 w5854 w5875 w5940 w6005 w6070 w6135 w6172 w6200 w6228 w6258 w6328 w6453 w6485 w6544 w6603 w6662 w6737 w6741 w6761 w6788 w6804 w6825 w6852 w6879 w6906 w6933 w6960 w6995 w7030 w7065 w7105 w7125 w7140 w7155 w7170 w7185 w7200 w7215 w7230 w7261 w7290 w7314 w7356 w7390 w7418 w7444 w7472 w7492 w7507 w7527 w7596 w7930 w7965 w7985 w8005 w8020 w8040 w8060 w8080 w8095 w8115 w8135 w8155 w8170 w8190 w8210 w8230 w8245 w8265 w8285 w8305]
      tunnel: w68 -> [w136 w1480 w1556 w1640 w1707 w1774 w1806 w1813 w1939 w2126 w2158 w2190 w2222 w2256 w2290 w2324 w2361 w2373 w2400 w2540 w2593 w3146 w3212 w3573 w3580 w3670 w4397 w4578 w4767 w4944 w5144 w5153 w5162 w5341 w5464 w5587 w5713 w5835 w5855 w5874 w5939 w6004 w6069 w6133 w6170 w6198 w6226 w6257 w6327 w6452 w6484 w6543 w6602 w6661 w6736 w6740 w6760 w6787 w6803 w6824 w6851 w6878 w6905 w6932 w6959 w6994 w7029 w7064 w7104 w7124 w7139 w7154 w7169 w7184 w7199 w7214 w7229 w7260 w7289 w7313 w7355 w7389 w7417 w7443 w7471 w7491 w7506 w7526 w7597 w7929 w7964 w7984 w8004 w8019 w8039 w8059 w8079 w8094 w8114 w8134 w8154 w8169 w8189 w8209 w8229 w8244 w8264 w8284 w8304]
      tunnel: [w107 w1485 w1556 w1578 w1645 w1712 w1793 w1820 w1946 w2037 w2145 w2177 w2209 w2247 w2281 w2315 w2352 w2373 w2385 w2505 w2600 w3060 w3206 w3571 w3577 w3696 w4391 w4572 w4761 w4945 w5145 w5153 w5155 w5337 w5474 w5598 w5723 w5833 w5853 w5873 w5938 w6003 w6068 w6134 w6171 w6199 w6227 w6256 w6326 w6450 w6483 w6542 w6601 w6660 w6729 w6739 w6759 w6786 w6802 w6823 w6850 w6877 w6904 w6931 w6958 w6993 w7028 w7063 w7103 w7123 w7138 w7153 w7168 w7183 w7198 w7213 w7228 w7245 w7287 w7312 w7354 w7388 w7416 w7442 w7454 w7474 w7494 w7510 w7534 w7931 w7950 w7967 w7987 w8007 w8025 w8042 w8062 w8082 w8098 w8117 w8137 w8157 w8173 w8192 w8212 w8232 w8248 w8267 w8287] -> w67
      tunnel: [w133 _ _ _ _ _ _ _ _ _ _ _ _ _ _ _ _ _ _ _ _ _ _ _ _ _ _ _ _ _ _ _ _ _ _ _ _ _ _ _ _ _ _ _ _ _ _ _ _ _ _ _ _ _ _ _ _ _ _ _ _ _ _ _ _ _ _ _ _ _ _ _ _ _ _ _ _ _ _ _ _ _ _ _ _ _ _ _ _ _ _ _ _ _ _ _ _ _ _ _ _ _ _ _ _ _ _ _ _] -> w66
      tunnel: w48 -> [_ _ _ _ _ _ _ _ _ _ _ _ _ _ _ _ _ _ _ _ _ _ w3205 _ _ _ w4396 w4576 _ w4949 _ _ w5160 w5350 w5473 w5597 w5722 _ _ _ _ _ _ _ _ _ _ _ _ _ _ _ _ _ _ _ _ _ _ _ _ _ _ _ _ _ _ _ _ _ _ _ _ _ _ _ _ _ _ _ _ _ _ _ _ _ _ _ _ _ _ _ _ _ _ _ _ _ _ _ _ _ _ _ _ _ _ _ _]
      tunnel: w63 -> [_ _ _ _ _ _ _ _ _ _ _ _ _ _ _ _ _ _ _ _ _ _ w3204 _ _ _ w4395 _ w4765 w4948 _ _ w5159 w5349 w5472 w5596 w5721 _ _ _ _ _ _ _ _ _ _ _ _ _ _ _ _ _ _ _ _ _ _ _ _ _ _ _ _ _ _ _ _ _ _ _ _ _ _ _ _ _ _ _ _ _ _ _ _ _ _ _ _ _ _ _ _ _ _ _ _ _ _ _ _ _ _ _ _ _ _ _ _]
      tunnel: w62 -> [_ _ _ _ _ _ _ _ _ _ _ _ _ _ _ _ _ w2366 _ _ _ _ _ _ _ _ _ _ _ _ _ _ _ _ _ _ _ _ _ _ _ _ _ _ _ _ _ _ _ _ _ _ _ _ _ _ _ _ _ _ _ _ _ _ _ _ _ _ _ _ _ _ _ _ _ _ _ _ _ _ _ _ _ _ _ _ _ _ _ _ _ _ _ _ _ _ _ _ _ _ _ _ _ _ _ _ _ _ _]
      tunnel: [w108 w1486 w1557 w1579 w1646 w1713 w1784 w1821 w1947 w2039 w2136 w2168 w2200 w2224 w2258 w2292 w2329 w2365 w2384 w2506 w2604 w3061 w3203 w3570 w3576 w3695 w4392 w4573 w4762 w4946 w5146 w5154 w5156 w5338 w5471 w5595 w5720 w5832 w5852 w5872 w5937 w6002 w6067 w6132 w6169 w6197 w6225 w6254 w6324 w6451 w6482 w6541 w6600 w6659 w6718 w6738 w6758 w6778 w6801 w6822 w6849 w6876 w6903 w6930 w6957 w6992 w7027 w7062 w7096 w7119 w7134 w7149 w7164 w7179 w7194 w7209 w7224 w7244 w7262 w7299 w7323 w7371 w7402 w7430 w7453 w7473 w7493 w7508 w7535 w7932 w7946 w7966 w7986 w8006 w8023 w8041 w8061 w8081 w8096 w8116 w8136 w8156 w8171 w8191 w8211 w8231 w8246 w8266 w8286] -> w55
